vi "MakeThetaLabels.vi"(1 "AxisBounds":T1={"Min"={"Auto"=TRUE, "Value"=0.0}, "Max"={"Auto"=TRUE, "Value"=0.0}}, 2 "ticsAndGrids":T3={"tics"={"ticMin"=0.0, "ticStep"=0.0, "ticMax"=0.0, "minorDivsPerMajor"=2, "ticSpacing"=enum."Auto Tics", "ticPosition"=enum."Inside, no mirror"}, "Grids"={"Gridlines"=enum."Major grid", "Zeroaxis"=enum."No zero axis"}, "Mapping"=enum."Lin"}) -> (0 "resulting string":string)   [LabVIEW 2015]
uses:
  ticsAndGrids.ctl
  tics.ctl
  grids.ctl
  minAndMax.ctl
  AutoManualNumber.ctl
panel:
  out "String":string="do for [jip = 0:7]{\nthetaer = jip*45;\ntexter = sprintf(\"%5.0f\",thetaer)\nset_label(x,text) = sprintf(\"set label '%s%s' at (-0.85*cos(90+%f)), (0.85*sin(90+%f)) center\", texter, \"$^{o}$\", thetaer, thetaer) #this places a label on the outside\neval set_label(thetaer,texter)\n}\n\n# set Cardinal Direction Arrow Properties\narowlength = 0.25\narowhalflength = arowlength/2\narowctrptx = -1\narowctrpty = -0.375\narowlftptx = arowctrptx - arowhalflength\narowrghtptx = arowctrptx + arowhalflength\narowtoppty = arowctrpty + arowhalflength\narowbotpty = arowctrpty - arowhalflength\nset arrow from arowctrptx,arowbotpty to arowctrptx,arowtoppty\nset arrow from arowlftptx,arowctrpty to arowrghtptx,arowctrpty nohead\nset label \"N\" at arowctrptx,arowtoppty+0.05 center"
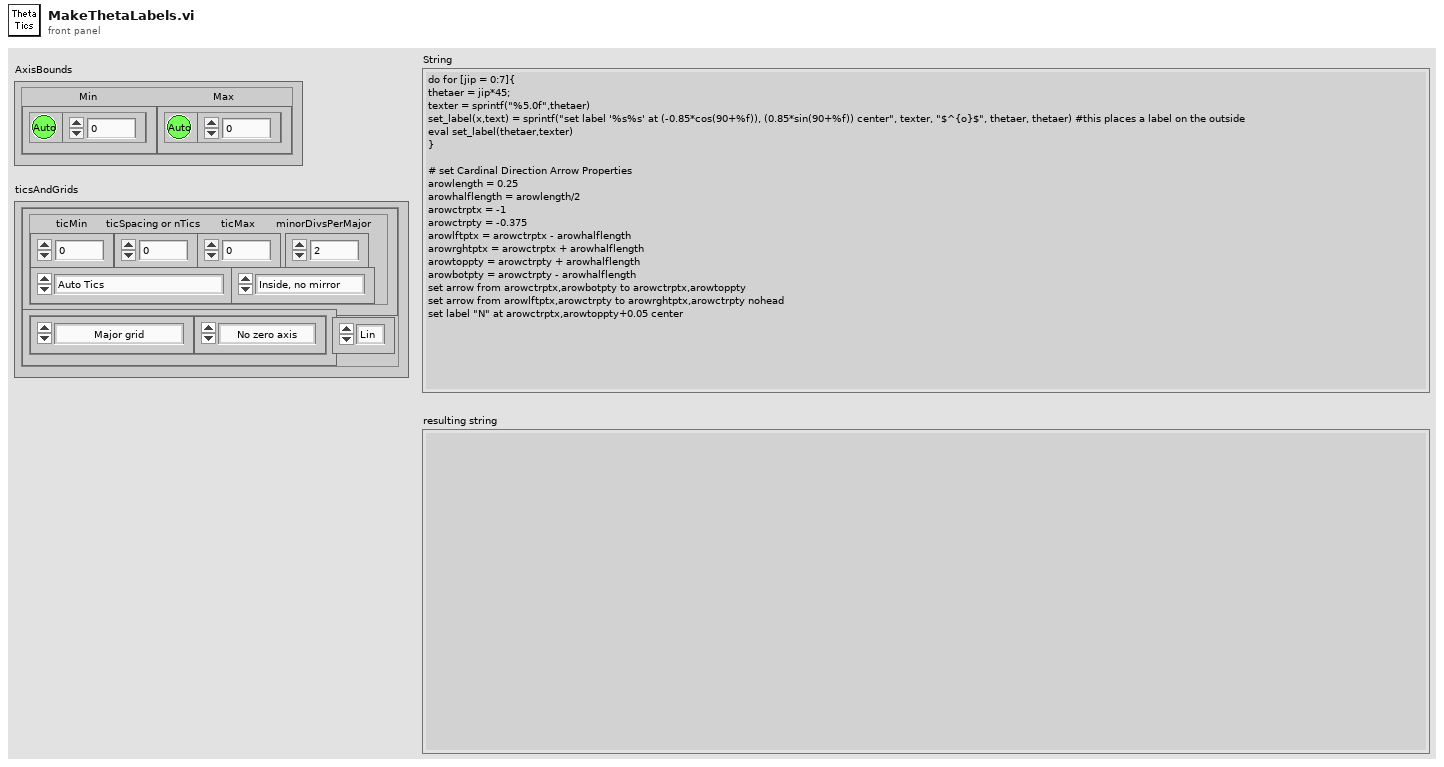
[diagram p1: front panel]
types:
  T1 = typedef "minAndMax.ctl" = cluster{"Min":T2, "Max":T2}
  T2 = typedef "AutoManualNumber.ctl" = cluster{"Auto":bool, "Value":dbl}
  T3 = typedef "ticsAndGrids.ctl" = cluster{"tics":T4, "Grids":T5, "Mapping":enum8{"Lin", "Log"}}
  T4 = typedef "tics.ctl" = cluster{"ticMin":dbl, "ticStep":dbl, "ticMax":dbl, "minorDivsPerMajor":i32, "ticSpacing":enum16{"Auto Tics", "Fixed spacing", "Fixed Minimum and Spacing", "Start, Spacing and Maximum", "Approx n Tics (rounded)"}, "ticPosition":enum16{"Inside, no mirror", "Inside, mirrored", "Outside, no mirror", "Outside, mirrored", "Invisible"}}
  T5 = typedef "grids.ctl" = cluster{"Gridlines":enum16{"No grids", "Major grid", "Minor grid", "Major and Minor"}, "Zeroaxis":enum16{"No zero axis", "Show zero axis"}}
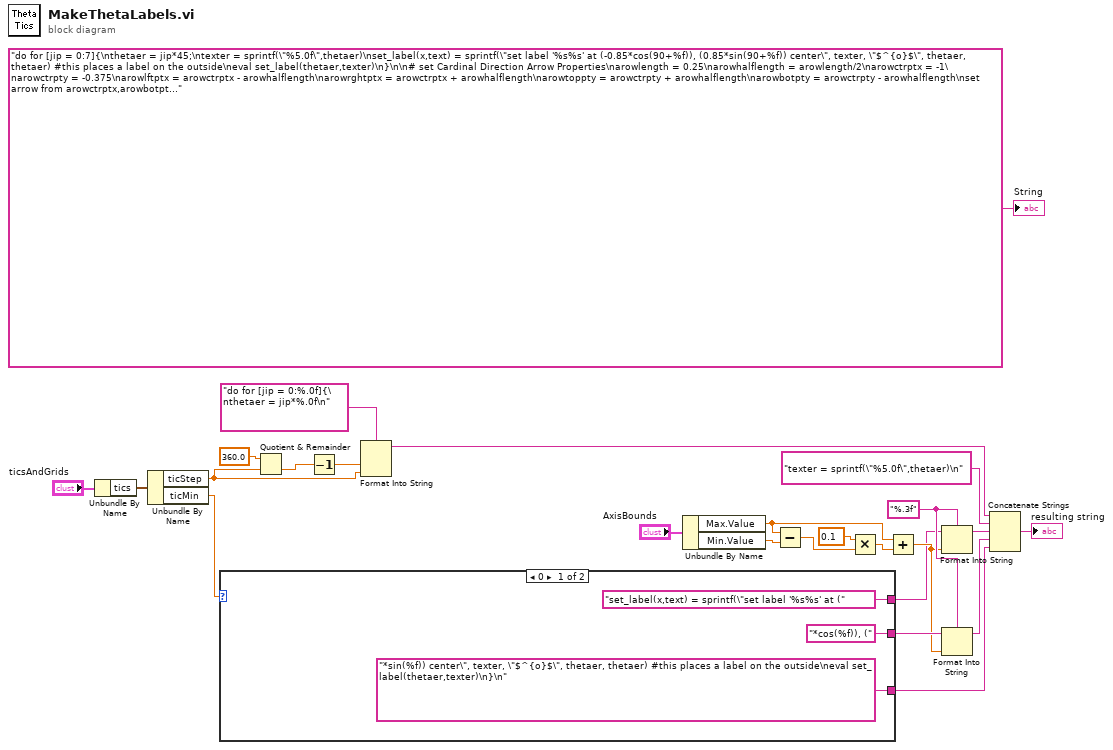
[diagram p0: block diagram]
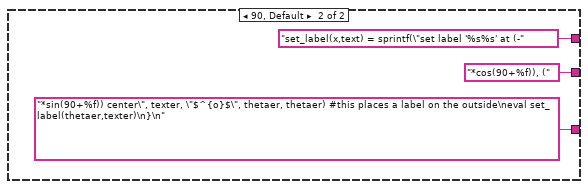
[diagram p2: hidden frame]
diagram:
  w4 = "%.3f" ("format string")
  n1 = Unbundle By Name("ticsAndGrids") -> ("tics"=w25:T4)
  n2 = Unbundle By Name(w25) -> ("ticStep"=w19:dbl, "ticMin"=w2:dbl)
  n3 = case shown="0" w2 {
    tunnel: ["*sin(%f)) center\", texter, \"$^{o}$\", thetaer, thetaer) #this places a label on the outside\neval set_label(thetaer,texter)\n}\n" "*sin(90+%f)) center\", texter, \"$^{o}$\", thetaer, thetaer) #this places a label on the outside\neval set_label(thetaer,texter)\n}\n"] -> w13
    tunnel: ["*cos(%f)), (" "*cos(90+%f)), ("] -> w5
    tunnel: ["set_label(x,text) = sprintf(\"set label '%s%s' at (" "set_label(x,text) = sprintf(\"set label '%s%s' at (-"] -> w1
    frame 0 {
    }
    frame 90, Default {
    }
  }
  n4 = Quotient & Remainder(x=360.0, y=w19) -> (floor(x/y)=w23:dbl)  [unwired: 1 out]
  n5 = Decrement(x=w23) -> (x-1=w20:dbl)
  n6 = Format Into String(format string="do for [jip = 0:%.0f]{\nthetaer = jip*%.0f\n", w20, w19) -> (resulting string=w17:string)  [unwired: 2 in, 1 out]
  n7 = Unbundle By Name("AxisBounds") -> ("Max.Value"=w6:dbl, "Min.Value"=w10:dbl)
  n8 = Subtract(x=w6, y=w10) -> (x-y=w9:dbl)
  n9 = Multiply(x=0.1, y=w9) -> (x*y=w7:dbl)
  n10 = Add(x=w6, y=w7) -> (x+y=w3:dbl)
  n11 = Format Into String(format string=w4, initial string=w1, w3) -> (resulting string=w15:string)  [unwired: 1 in, 1 out]
  n12 = Format Into String(format string=w4, initial string=w5, w3) -> (resulting string=w14:string)  [unwired: 1 in, 1 out]
  n13 = Concatenate Strings(w17, "texter = sprintf(\"%5.0f\",thetaer)\n" ("string"), w15, w14, w13) -> (→"resulting string":string)
  "String" <- "do for [jip = 0:7]{\nthetaer = jip*45;\ntexter = sprintf(\"%5.0f\",thetaer)\nset_label(x,text) = sprintf(\"set label '%s%s' at (-0.85*cos(90+%f)), (0.85*sin(90+%f)) center\", texter, \"$^{o}$\", thetaer, thetaer) #this places a label on the outside\neval set_label(thetaer,texter)\n}\n\n# set Cardinal Direction Arrow Properties\narowlength = 0.25\narowhalflength = arowlength/2\narowctrptx = -1\narowctrpty = -0.375\narowlftptx = arowctrptx - arowhalflength\narowrghtptx = arowctrptx + arowhalflength\narowtoppty = arowctrpty + arowhalflength\narowbotpty = arowctrpty - arowhalflength\nset arrow from arowctrptx,arowbotpty to arowctrptx,arowtoppty\nset arrow from arowlftptx,arowctrpty to arowrghtptx,arowctrpty nohead\nset label \"N\" at arowctrptx,arowtoppty+0.05 center"
